vi "dfd_Direct IIR I Transposed Normalization.vi"(7 "scale type":T1, 9 "coefficients b":dbl[](array[numeric]) format="%.2f", 10 "coefficients a":dbl[](array[numeric]) format="%.2f", 11 "x":dbl[](array[numeric])) -> (2 "norm":dbl[](array[numeric]) format="%.2f", 3 "y":dbl[](array[numeric]))   [LabVIEW 2017, in "NI_DigFilter_FXP.lvlib"]
uses:
  <vilib>/addons/Digital Filter Design/NI_DigFilter_FXP.lvlib
  <vilib>/addons/Digital Filter Design/_Objects.llb/DFD Coef Norm Type.ctl
  <vilib>/addons/Digital Filter Design/NI_DigFilterLicensed.lvlib
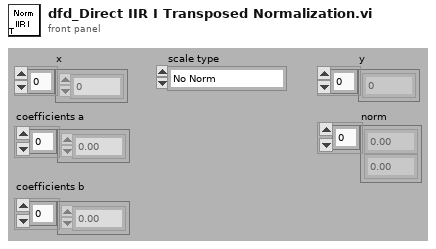
[diagram p1: front panel]
types:
  T1 = typedef "NI_DigFilterLicensed.lvlib/DFD Coef Norm Type.ctl" = enum16{"No Norm", "Time Domain 1-Norm", "Time Domain 2-Norm", "Time Domain Inf-Norm"}
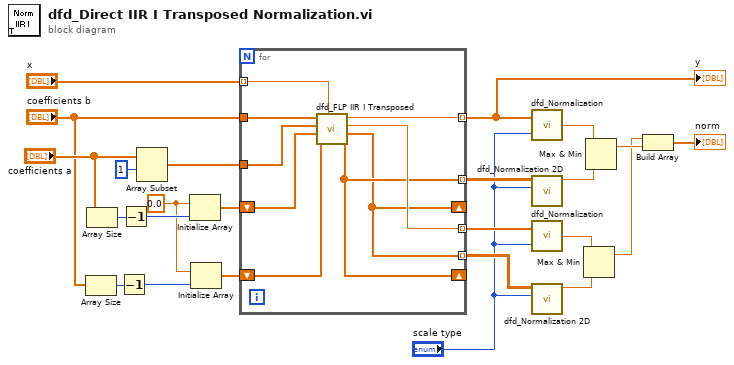
[diagram p0: block diagram]
diagram:
  w13 = 0.0 ("element")
  n1 = Array Size(array="coefficients b") -> (size(s)=w21:i32)
  n2 = Array Size(array="coefficients a") -> (size(s)=w22:i32)
  n3 = Decrement(x=w21) -> (x-1=w15:i32)
  n4 = Decrement(x=w22) -> (x-1=w14:i32)
  n5 = Array Subset(array="coefficients a", index=1) -> (w19:dbl[])  [unwired: 1 in]
  n6 = Initialize Array(w13, w14) -> (w18:dbl[])
  n7 = Initialize Array(w13, w15) -> (w24:dbl[])
  n8 = for {
    shift-right: [w27] -> _
    shift-left: w24 -> [w29]
    tunnel: [w31] -> w9 mode=indexing
    tunnel: w19 -> [w33]
    shift-right: [w26] -> _
    shift-left: w18 -> [w28]
    tunnel: "coefficients b" -> [w32]
    tunnel: [w30] -> w8 mode=indexing
    tunnel: [w27] -> w11 mode=indexing
    tunnel: [w26] -> w10 mode=indexing
    tunnel: "x" -> [w25] mode=indexing
    (unwired) 0.0 ("element")
    n9 = call <vilib>:"dfd_FLP IIR I Transposed.vi"("x"=w25, "y states in"=w29, "x states in"=w28, "coefficients a"=w33, "coefficents b"=w32) -> ("y states out"=w27:dbl[], "x states out"=w26:dbl[], "w"=w30:dbl, "y"=w31:dbl)  [unwired: 3 out]
  }
  "y" <- w9
  n10 = call <vilib>:"dfd_Normalization.vi"("scale type"="scale type", "h(n)"=w9) -> ("norm"=w6:dbl)
  n11 = call <vilib>:"dfd_Normalization 2D.vi"("scale type"="scale type", "2D Array (col-major)"=w11) -> ("max norm"=w5:dbl)  [unwired: 1 in, 8 out]
  n12 = call <vilib>:"dfd_Normalization.vi"("scale type"="scale type", "h(n)"=w8) -> ("norm"=w3:dbl)
  n13 = call <vilib>:"dfd_Normalization 2D.vi"("scale type"="scale type", "2D Array (col-major)"=w10) -> ("max norm"=w2:dbl)  [unwired: 1 in, 8 out]
  n14 = Max & Min(x=w3, y=w2) -> (max(x,y)=w1:dbl)  [unwired: 1 out]
  n15 = Max & Min(x=w6, y=w5) -> (max(x,y)=w4:dbl)  [unwired: 1 out]
  n16 = Build Array(w1, w4) -> (→"norm":dbl[])
